vi "make_headers.vi"(5 "Content-Type":string, 8 "Error in":errorcluster, 11 "Device In":T1) -> (0 "Error Out":errorcluster, 3 "Device Out":T1)   [LabVIEW 2019]
uses:
  SHA256/SHA256.lvlib
  <vilib>/Utility/SMTP/NI_SMTPEmail.lvlib
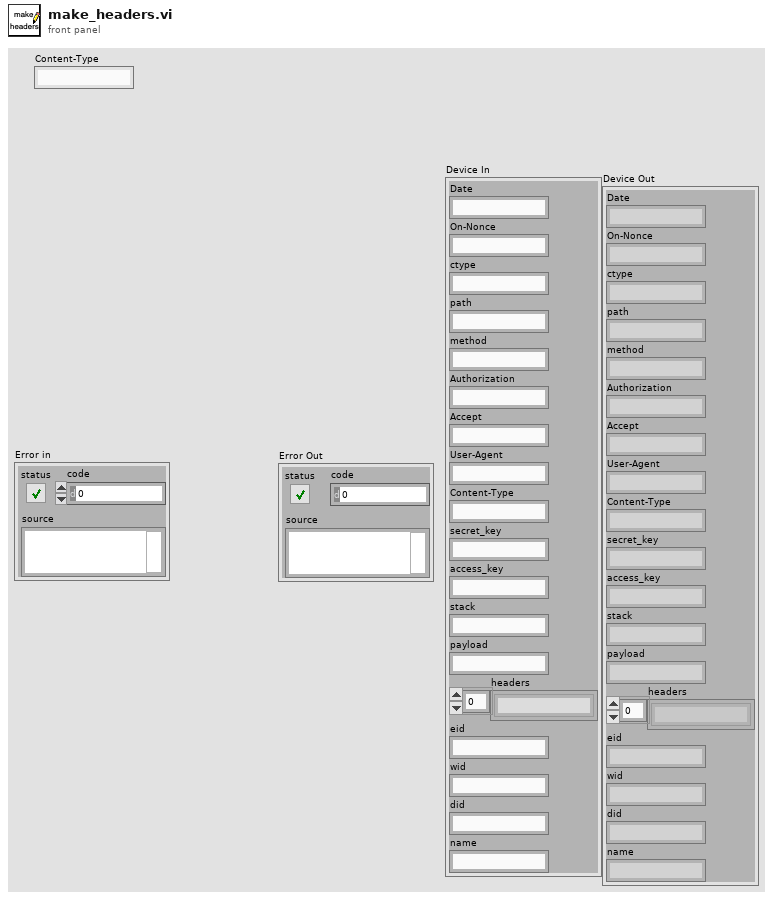
[diagram p1: front panel]
types:
  T1 = cluster{"Date":string, "On-Nonce":string, "ctype":string, "path":string, "method":string, "Authorization":string, "Accept":string, "User-Agent":string, "Content-Type":string, "secret_key":string, "access_key":string, "stack":string, "payload":string, "headers":string[], "eid":string, "wid":string, "did":string, "name":string}
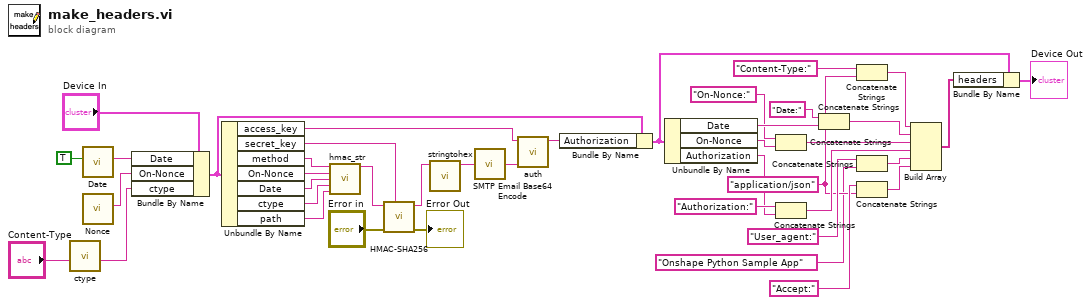
[diagram p0: block diagram]
diagram:
  w4 = "application/json" ("Content-Type")
  n1 = call "ctype.vi"("Content-Type"="Content-Type") -> ("ctype"=w40:string)  [unwired: 10 in]
  n2 = call "Date.vi"("UTC format"=TRUE) -> ("date/time string"=w29:string)  [unwired: 10 in]
  n3 = call "Nonce.vi"() -> ("Nonce"=w28:string)  [unwired: 11 in]
  n4 = Bundle By Name(cluster="Device In", "Date"=w29, "On-Nonce"=w28, "ctype"=w40) -> (w22:T1)
  n5 = Unbundle By Name(w22) -> ("access_key"=w30:string, "secret_key"=w31:string, "method"=w39:string, "On-Nonce"=w38:string, "Date"=w37:string, "ctype"=w35:string, "path"=w36:string)
  n6 = call "hmac_str.vi"("Method"=w39, "Nonce"=w38, "Date"=w37, "ctype"=w35, "path"=w36) -> ("hmac_str"=w34:string)  [unwired: 10 in]
  n7 = call "HMAC-SHA256.vi"("Key"=w31, "error In"="Error in", "String to Encode"=w34) -> ("error Out"=→"Error Out":errorcluster, "Hash String"=w27:string)  [unwired: 7 in]
  n8 = call "stringtohex.vi"("Hash String"=w27) -> ("string"=w26:string)  [unwired: 10 in]
  n9 = call "SMTP Email Base64 Encode.vi"("Normal String"=w26) -> ("Base64 String"=w33:string)  [unwired: 1 in]
  n10 = call "auth.vi"("signature"=w33, "access_key"=w30) -> ("auth"=w32:string)  [unwired: 9 in]
  n11 = Bundle By Name(cluster=w22, "Authorization"=w32) -> (w21:T1)
  n12 = Unbundle By Name(w21) -> ("Date"=w18:string, "On-Nonce"=w16:string, "Authorization"=w14:string)
  n13 = Concatenate Strings("On-Nonce:" ("string"), w16) -> (w9:string)
  n14 = Concatenate Strings("Authorization:" ("string"), w14) -> (w8:string)
  n15 = Concatenate Strings("Date:" ("string"), w18) -> (w10:string)
  n16 = Concatenate Strings("Content-Type:" ("string"), w4) -> (w11:string)
  n17 = Concatenate Strings("User_agent:" ("string"), "Onshape Python Sample App" ("User-Agent")) -> (w7:string)
  n18 = Concatenate Strings("Accept:" ("string"), w4) -> (w6:string)
  n19 = Build Array(w11, w10, w9, w8, w7, w6) -> (w5:string[])
  n20 = Bundle By Name(cluster=w21, "headers"=w5) -> (→"Device Out":T1)
